vi "STM Command Based Example - Server.vi"() -> ()   [LabVIEW 2020]
doc: "This example demonstrates how to use STM with TCP to implement a command based communications application. \n\nThe server receives messages from the client on the type of signals to generate (frequency, FFT window type) and then sends time domain and spectral data to the client.\n\nThe server must be started first.\n\nCopyright 2015, 2016, 2017 National Instruments Corporation\n\nLicensed under the Apache License, Version 2.0 (the \"License\"); you may not use this file except in compliance with the License.\n\n You may obtain a copy of the License at\n\n http://www.apache.org/licenses/LICENSE-2.0\n\nUnless required by applicable law or agreed to in writing, software distributed under the License is distributed on an \"AS IS\" BASIS, WITHOUT WARRANTIES OR CONDITIONS OF ANY KIND, either express or implied.\n\nSee the License for the specific language governing permissions and limitations under the License."
uses:
  <vilib>/NI/STM/SubVIs/MetaDataElement.ctl
  <vilib>/NI/STM/TCP/TCP Read Options.ctl
  <vilib>/NI/STM/TCP/Write Meta Data (TCP Ref).vi
  <vilib>/NI/STM/TCP/Get Connection Reference (TCP).vi
  <vilib>/NI/STM/TCP/Write Meta Data (TCP Clst).vi
  <vilib>/measure/maspectr.llb/FFT Power Spectrum for 1 Chan.vi
  <vilib>/NI/STM/TCP/Write Message (TCP).vi
  <vilib>/NI/STM/TCP/Read Message (TCP).vi
  <vilib>/measure/NI_MAPro.lvlib
  <vilib>/measure/NI_MABase.lvlib
  <vilib>/NI/STM/NI STM.lvlib
panel:
  out "Window":T1(ring)
  out "error out":errorcluster
  in  "stop":bool
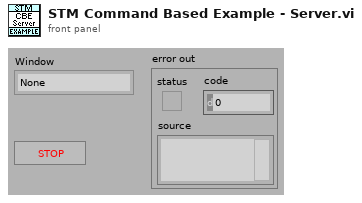
[diagram p1: front panel]
types:
  T1 = enum16{"None ", "Hanning", "Hamming", "Blackman-Harris", "Exact Blackman", "Blackman", "Flat Top", "4 Term B-Harris ", "7 Term B-Harris", "Low Sidelobe"}
  T2 = typedef "NI STM.lvlib/MetaDataElement.ctl" = string
  T3 = typedef "NI STM.lvlib/TCP Connection Info.ctl" = cluster{"connection ID":refnum<k5>, "meta data":T2[]}
  T4 = typedef "Command Based Example Queue Refs.ctl" = cluster{"Data Queue":refnum<queue>, "Frequency Queue":refnum<queue>}
  T5 = typedef "NI STM.lvlib/TCP Read Options.ctl" = cluster{"ignore timeout error":bool, "timeout ms (1000)":i32}
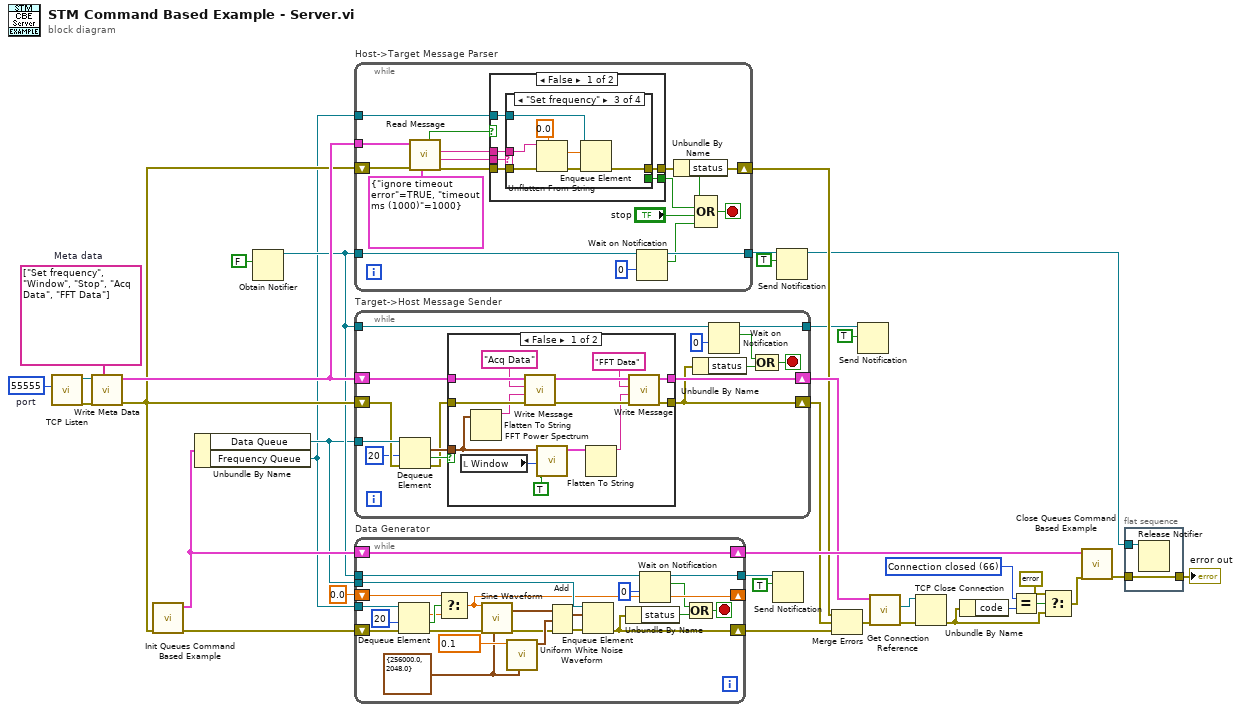
[diagram p0: block diagram]
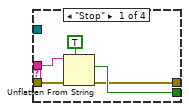
[diagram p3: hidden frame]
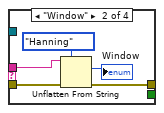
[diagram p4: hidden frame]
diagram:
  w6 = 66 items=["No Error", "Argument Error", "Memory Full", "Out of Zone", "End of File", "File Already Open", "Generic File IO Error", "File Not Found", "File Permission Error", "Disk Full", "Duplicate Path", "Too Many Files Open", "Not Enabled", "Resource File Not Found", "Cannot Add Resource", "Resource Not Found", "Image Not Found", "Image Memory Error", "Pen Does Not Exist", "Config Bad Type", "Config Token Not Found", "Config Parse Error", "Config Memory Error", "Bad External Code Format", "Bad External Code Offset", "External Code Not Present", "Null Window", "Destroy Window Mixup", "Null Menu", "Print Aborted", "Bad Print Record", "Print Driver Error", "Windows Error During Print", "Memory Error During Print", "Print Dialog Error", "Generic Print Error", "Invalid Device Refnum", "Device Not Found", "Device Parameter Error", "Device Unit Error", "Can't Open Device", "Device Call Aborted", "Generic Error", "Cancelled By User", "Object ID Too Low", "Object ID Too High", "Object Not In Heap", "Unknown Heap", "Bad DefProc ID", "DefProc Not In Table", "Message Out Of Range", "Null Method", "Unknown Message", "Manager Call Not Supported", "Bad address", "Connection In progress", "Connection timed out", "Connection is already in progress", "Network attribute not supported", "Network error", "Address in use", "System out of memory", "Connection aborted", "Connection refused", "Connection is not connected", "Connection is already connected", "Connection closed", "Initialize error (interapplication manager)", "Bad occurrence", "Wait on unbound occurrence handler", "Occurrence queue overflow", "Bad path", "Semaphore not signaled", "Unrecognized type (interapplication manager)"] ("1st Error to Convert")
  w20 = T2[] ["Set frequency", "Window", "Stop", "Acq Data", "FFT Data"]  # Meta data
  w36 = u16 55555  # port
  n1 = call <vilib>:"TCP Listen.vi"("port"=w36) -> ("error out"=w34:errorcluster, "connection ID"=w35:refnum<k5>)  [unwired: 3 in, 6 out]
  n2 = call-poly <vilib>:"Write Meta Data.vi"("meta data"=w20, "error in"=w34, "connection ID"=w35) -> ("error out"=w32:errorcluster, "connection info out"=w33:T3)  [unwired: 2 in, 5 out]
  n3 = call "Init Queues Command Based Example.vi"("error in (no error)"=w32) -> ("error out"=w30:errorcluster, "Queue Refs"=w29:T4)  [unwired: 9 out]
  n4 = Unbundle By Name(w29) -> ("Data Queue"=w2:refnum<queue>, "Frequency Queue"=w1:refnum<queue>)
  n5 = Obtain Notifier(notification data type=FALSE) -> (notifier out=w14:refnum<notifier>)  [unwired: 3 in, 2 out]
  n6 = while "Host->Target Message Parser" {
    tunnel: w33 -> [w53]
    tunnel: w1 -> [w48]
    shift-right: [w43] -> w22
    shift-left: w32 -> [w52]
    tunnel: w14 -> [w45]
    tunnel: [w40] -> w18
    stop <- w41 stop-if-true
    n7 = call-poly <vilib>:"Read Message.vi"("options"=T5 {"ignore timeout error"=TRUE, "timeout ms (1000)"=1000} ("Options"), "error in"=w52, "connection info in"=w53) -> ("error out"=w47:errorcluster, "name"=w51:T2, "data string"=w50:string, "timed out?"=w49:bool)  [unwired: 2 in, 3 out]
    n8 = case shown="False" w49 {
      tunnel: w51 -> [w55 _]
      tunnel: w50 -> [w59 _]
      tunnel: w48 -> [w58 _]
      tunnel: w47 -> [w57 w78]
      tunnel: [w56 w78] -> w43
      tunnel: [w54 _] -> w38
      frame False {
        n9 = case shown="\"Set frequency\"" w55 {
          tunnel: w59 -> [w63 w67 w73 _]
          tunnel: w58 -> [_ _ w76 _]
          tunnel: w57 -> [w62 w66 w72 w77]
          tunnel: [w60 w65 w70 w77] -> w56
          tunnel: [w61 _ _ _] -> w54
          frame "Stop" {
            n10 = Unflatten From String(type=TRUE, binary string=w63, error in (no error)=w62) -> (value=w61:bool, error out=w60:errorcluster)  [unwired: 1 in, 2 out]
          }
          frame "Window" {
            n11 = Unflatten From String(type=T1."Hanning" ("window"), binary string=w67, error in (no error)=w66) -> (value=→"Window":T1, error out=w65:errorcluster)  [unwired: 1 in, 2 out]
          }
          frame "Set frequency" {
            n12 = Unflatten From String(type=0.0, binary string=w73, error in (no error)=w72) -> (value=w74:dbl, error out=w71:errorcluster)  [unwired: 1 in, 2 out]
            n13 = Enqueue Element(queue=w76, element=w74, error in (no error)=w71) -> (error out=w70:errorcluster)  [unwired: 3 out]
          }
          frame Default {
          }
        }
      }
      frame True {
      }
    }
    n14 = Wait on Notification(notifier=w45, timeout in ms (-1)=0) -> (notifier out=w40:refnum<notifier>, notification=w39:bool)  [unwired: 2 in, 2 out]
    n15 = Unbundle By Name(w43) -> ("status"=w42:bool)
    n16 = Compound Arithmetic op=OR(w42, w38, "stop", w39) -> (w41:bool)
  }
  n17 = while "Target->Host Message Sender" {
    tunnel: w2 -> [w91]
    shift-right: [w83] -> w24
    shift-left: w32 -> [w88]
    shift-right: [w92] -> w27
    shift-left: w33 -> [w93]
    tunnel: w14 -> [w84]
    tunnel: [w79] -> w15
    stop <- w80 stop-if-true
    n18 = Dequeue Element(queue=w91, timeout in ms (-1)=20, error in (no error)=w88) -> (element=w90:waveform(dbl), timed out?=w89:bool, error out=w87:errorcluster)  [unwired: 1 out]
    n19 = case shown="False" w89 {
      tunnel: w93 -> [w107 w109]
      tunnel: w87 -> [w106 w108]
      tunnel: [w102 w109] -> w92
      tunnel: [w104 w108] -> w83
      tunnel: w90 -> [w94 _]
      frame False {
        n20 = local read "Window"() -> (w96:T1)
        n21 = Flatten To String(anything=w94) -> (data string=w99:string)  [unwired: 1 in, 4 out]
        n22 = call-poly <vilib>:"Write Message.vi"("error in"=w106, "data"=w99, "name"="Acq Data" ("Name"), "connection info in"=w107) -> ("error out"=w101:errorcluster, "connection info out"=w103:T3)  [unwired: 1 in, 5 out]
        n23 = call-poly <vilib>:"FFT Power Spectrum.vi"("dB On (F)"=TRUE, "window"=w96, "time signal"=w94) -> ("power spectrum"=w98:cluster{"f0":dbl, "df":dbl, "magnitude":dbl[]})  [unwired: 3 in, 5 out]
        n24 = Flatten To String(anything=w98) -> (data string=w97:string)  [unwired: 1 in, 4 out]
        n25 = call-poly <vilib>:"Write Message.vi"("error in"=w101, "data"=w97, "name"="FFT Data" ("Name"), "connection info in"=w103) -> ("error out"=w104:errorcluster, "connection info out"=w102:T3)  [unwired: 1 in, 5 out]
      }
      frame True {
      }
    }
    n26 = Unbundle By Name(w83) -> ("status"=w82:bool)
    n27 = Wait on Notification(notifier=w84, timeout in ms (-1)=0) -> (notifier out=w79:refnum<notifier>, notification=w81:bool)  [unwired: 2 in, 2 out]
    n28 = Compound Arithmetic op=OR(w81, w82) -> (w80:bool)
  }
  n29 = while "Data Generator" {
    tunnel: w2 -> [w133]
    tunnel: w1 -> [w132]
    shift-right: [w117] -> _
    shift-left: 0.0 -> [w119]
    shift-right: [w114] -> w23
    shift-left: w30 -> [w131]
    shift-right: [w124] -> w28
    shift-left: w29 -> [w124]
    tunnel: w14 -> [w115]
    tunnel: [w110] -> w12
    stop <- w111 stop-if-true
    w125 = cluster{"Fs":dbl, "#s":dbl} {"Fs"=256000.0, "#s"=2048.0} ("sampling info")
    n30 = Dequeue Element(queue=w132, timeout in ms (-1)=20, error in (no error)=w131) -> (element=w118:dbl, timed out?=w120:bool, error out=w130:errorcluster)  [unwired: 1 out]
    n31 = Select(t=w119, s=w120, f=w118) -> (s? t:f=w117:dbl)
    n32 = call <vilib>:"Sine Waveform.vi"("sampling info"=w125, "error in (no error)"=w130, "frequency"=w117) -> ("error out"=w123:errorcluster, "signal out"=w128:waveform(dbl))  [unwired: 4 in, 3 out]
    n33 = call <vilib>:"Uniform White Noise Waveform.vi"("sampling info"=w125, "amplitude"=0.1 ("Amplitude")) -> ("signal out"=w127:waveform(dbl))  [unwired: 3 in, 6 out]
    n34 = Add(1:w127, 2:w128, 4:w123) -> (0:w126:waveform(dbl), 3:w122:errorcluster)
    n35 = Enqueue Element(queue=w133, element=w126, error in (no error)=w122) -> (error out=w114:errorcluster)  [unwired: 3 out]
    n36 = Unbundle By Name(w114) -> ("status"=w113:bool)
    n37 = Wait on Notification(notifier=w115, timeout in ms (-1)=0) -> (notifier out=w110:refnum<notifier>, notification=w112:bool)  [unwired: 2 in, 2 out]
    n38 = Compound Arithmetic op=OR(w112, w113) -> (w111:bool)
  }
  n39 = Send Notification(notification=TRUE, notifier=w12) -> ()  [unwired: 1 in, 2 out]
  n40 = Send Notification(notification=TRUE, notifier=w18) -> (notifier out=w11:refnum<notifier>)  [unwired: 1 in, 1 out]
  n41 = Merge Errors(w22, w24, w23) -> (w21:errorcluster)
  n42 = Send Notification(notification=TRUE, notifier=w15) -> ()  [unwired: 1 in, 2 out]
  n43 = call-poly <vilib>:"Get Connection Reference.vi"("error in"=w21, "connection info in"=w27) -> ("error out"=w25:errorcluster, "connection ID out"=w26:refnum<k5>)  [unwired: 8 out]
  n44 = TCP Close Connection(connection ID=w26, error in (no error)=w25) -> (error out=w5:errorcluster)  [unwired: 2 out]
  n45 = Unbundle By Name(w5) -> ("code"=w8:i32)
  n46 = Equal?(x=w6, y=w8) -> (x = y?=w7:bool)
  n47 = Select(t=errorcluster {"status"=FALSE, "code"=0, "source"=""}, s=w7, f=w5) -> (s? t:f=w4:errorcluster)
  n48 = call "Close Queues Command Based Example.vi"("error in (no error)"=w4, "FIFOs In"=w28) -> ("error out"=w10:errorcluster)  [unwired: 9 out]
  n49 = flat-sequence {
    tunnel: w11 -> [w135]
    tunnel: w10 -> [w134]
    tunnel: [w134] -> w9
    frame #0 {
      n50 = Release Notifier(notifier=w135) -> ()  [unwired: 2 in, 3 out]
    }
  }
  "error out" <- w9
